vi "_PC_DataChrom_Mass2XIC.vi"(5 "ChromType":enum16{"TIC", "XIC"}(ring), 7 "Limit":T1, 8 "error in (no error)":errorcluster, 11 "File Path Array":path[](array[path])) -> (0 "error out":errorcluster, 1 "Information":string[](array[string]), 3 "DataArray":cluster{"X":dbl[], "Y":dbl[]}[](array[cluster]))   [LabVIEW 2018]
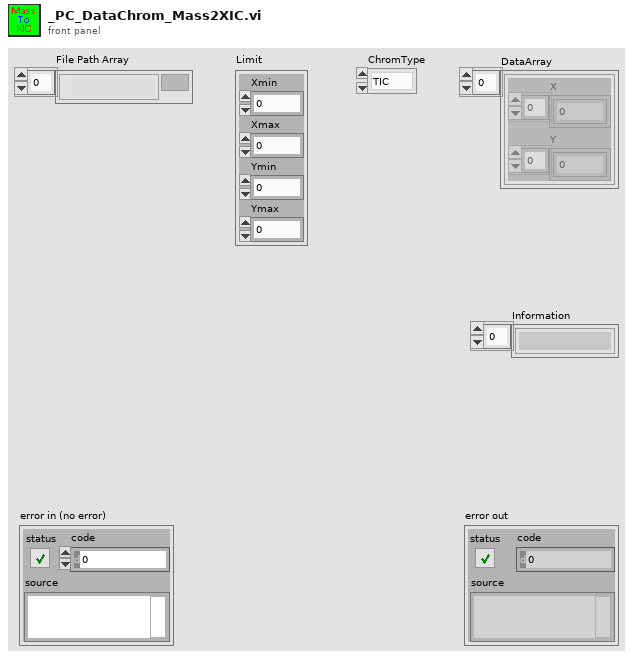
[diagram p1: front panel]
types:
  T1 = cluster{"Xmin":dbl, "Xmax":dbl, "Ymin":dbl, "Ymax":dbl}
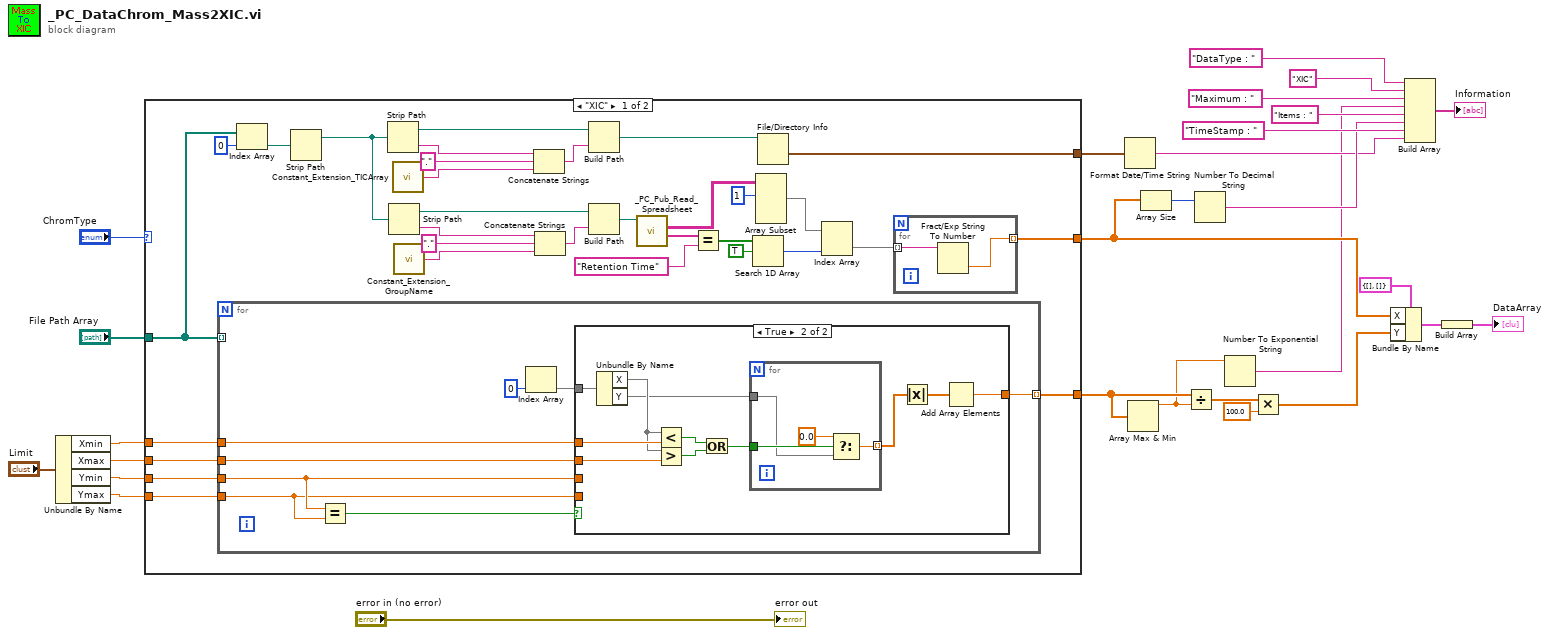
[diagram p0: block diagram]
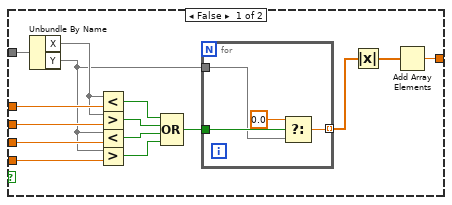
[diagram p2: hidden frame]
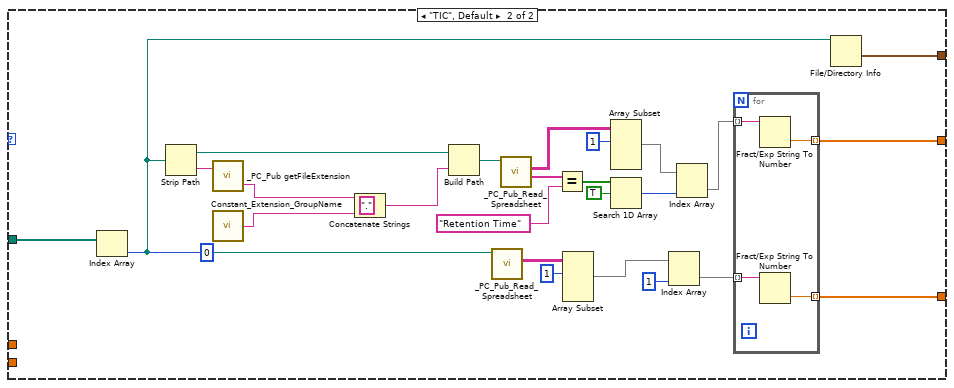
[diagram p3: hidden frame]
diagram:
  n1 = Unbundle By Name("Limit") -> ("Xmin"=w26:dbl, "Xmax"=w25:dbl, "Ymin"=w24:dbl, "Ymax"=w23:dbl)
  n2 = case shown="\"XIC\"" "ChromType" {
    tunnel: [w56 w109] -> w6
    tunnel: w26 -> [w60 _]
    tunnel: w25 -> [w59 _]
    tunnel: w24 -> [w58 _]
    tunnel: w23 -> [w57 _]
    tunnel: [w29 w110] -> w15
    tunnel: [w46 w113] -> w10
    tunnel: "File Path Array" -> [w55 w132]
    frame "XIC" {
      n3 = for {
        tunnel: [w69] -> w56 mode=indexing
        tunnel: w60 -> [w71]
        tunnel: w59 -> [w70]
        tunnel: w58 -> [w68]
        tunnel: w57 -> [w67]
        tunnel: w55 -> [_] mode=indexing
        n4 = Equal?(x=w68, y=w67) -> (x = y?=w66:bool)
        n5 = Index Array(index=0) -> (array=w65:cluster{"X":dbl[], "Y":sgl[]}[], element=w63)
        n6 = case shown="True" w66 {
          tunnel: w71 -> [w86 w101]
          tunnel: w70 -> [w85 w100]
          tunnel: w68 -> [w84 _]
          tunnel: w67 -> [w83 _]
          tunnel: [w73 w99] -> w69
          tunnel: w63 -> [w72 w91]
          frame False {
            n7 = Unbundle By Name(w72) -> ("X"=w82, "Y"=w76)
            n8 = Less?(x=w82, y=w86) -> (x < y?=w81:bool)
            n9 = Greater?(x=w82, y=w85) -> (0:w80:bool)
            n10 = Less?(x=w76, y=w84) -> (x < y?=w79:bool)
            n11 = Greater?(x=w76, y=w83) -> (0:w78:bool)
            n12 = Compound Arithmetic op=OR(w81, w80, w79, w78) -> (w77:bool)
            n13 = for {
              tunnel: w77 -> [w90]
              tunnel: w76 -> [w88]
              tunnel: [w87] -> w74 mode=indexing
              n14 = Select(t=0.0, s=w90, f=w88) -> (s? t:f=w87:dbl)
            }
            n15 = Absolute Value(x=w74) -> (abs(x)=w75:dbl[])
            n16 = Add Array Elements(numeric array=w75) -> (sum=w73:dbl)
          }
          frame True {
            n17 = Unbundle By Name(w91) -> ("X"=w98, "Y"=w94)
            n18 = Less?(x=w98, y=w101) -> (x < y?=w97:bool)
            n19 = Greater?(x=w98, y=w100) -> (0:w96:bool)
            n20 = Or(x=w97, y=w96) -> (x .or. y?=w95:bool)
            n21 = for {
              tunnel: w95 -> [w105]
              tunnel: w94 -> [w103]
              tunnel: [w102] -> w92 mode=indexing
              n22 = Select(t=0.0, s=w105, f=w103) -> (s? t:f=w102:dbl)
            }
            n23 = Absolute Value(x=w92) -> (abs(x)=w93:dbl[])
            n24 = Add Array Elements(numeric array=w93) -> (sum=w99:dbl)
          }
        }
      }
      n25 = Index Array(array=w55, index=0) -> (element=w53:path)
      n26 = Strip Path(path=w53) -> (stripped path=w33:path)  [unwired: 1 out]
      n27 = Strip Path(path=w33) -> (stripped path=w49:path, name=w50:string)
      n28 = Strip Path(path=w33) -> (stripped path=w32:path, name=w34:string)
      n29 = call "Constant_Extension_TICArray.vi"() -> ("Information Array Name String"=w51:string)
      n30 = call "Constant_Extension_GroupName.vi"() -> ("Group Name String"=w35:string)
      n31 = Concatenate Strings(w50, "." ("string"), w51) -> (w48:string)
      n32 = Concatenate Strings(w34, "." ("string"), w35) -> (w31:string)
      n33 = Build Path(base path=w49, name or relative path=w48) -> (appended path=w47:path)
      n34 = Build Path(base path=w32, name or relative path=w31) -> (appended path=w45:path)
      n35 = call "_PC_Pub_Read_Spreadsheet.vi"("file path (dialog if empty)"=w45) -> ("first row"=w39:string[], "all rows"=w38:string[][])  [unwired: 7 in, 2 out]
      n36 = Equal?(x=w39, y="Retention Time" ("String")) -> (x = y?=w43:bool[])
      n37 = Search 1D Array(1D array=w43, element=TRUE) -> (index of element=w37:i32)  [unwired: 1 in]
      n38 = Array Subset(array=w38, index (row)=1 ("index")) -> (w40:string[][])  [unwired: 3 in]
      n39 = File/Directory Info(path=w47) -> (last mod=w46:timestamp)  [unwired: 1 in, 6 out]
      n40 = Index Array(array=w40, index (col)=w37) -> (element=w30:string[])  [unwired: 1 in]
      n41 = for {
        tunnel: w30 -> [w62] mode=indexing
        tunnel: [w61] -> w29 mode=indexing
        n42 = Fract/Exp String To Number(string=w62) -> (number=w61:dbl)  [unwired: 3 in, 1 out]
      }
    }
    frame "TIC", Default {
      n43 = Index Array(array=w132, index=0) -> (element=w114:path)
      n44 = Strip Path(path=w114) -> (stripped path=w124:path, name=w126:string)
      n45 = call "_PC_Pub getFileExtension.vi"("Input"=w126) -> ("FileName"=w129:string)  [unwired: 1 in, 1 out]
      n46 = call "Constant_Extension_GroupName.vi"() -> ("Group Name String"=w127:string)
      n47 = Concatenate Strings(w129, "." ("string"), w127) -> (w125:string)
      n48 = Build Path(base path=w124, name or relative path=w125) -> (appended path=w123:path)
      n49 = call "_PC_Pub_Read_Spreadsheet.vi"("file path (dialog if empty)"=w114) -> ("all rows"=w108:string[][])  [unwired: 7 in, 3 out]
      n50 = call "_PC_Pub_Read_Spreadsheet.vi"("file path (dialog if empty)"=w123) -> ("first row"=w117:string[], "all rows"=w116:string[][])  [unwired: 7 in, 2 out]
      n51 = Equal?(x=w117, y="Retention Time" ("String")) -> (x = y?=w121:bool[])
      n52 = Array Subset(array=w108, index (row)=1 ("index")) -> (w107:string[][])  [unwired: 3 in]
      n53 = Array Subset(array=w116, index (row)=1 ("index")) -> (w118:string[][])  [unwired: 3 in]
      n54 = Search 1D Array(1D array=w121, element=TRUE) -> (index of element=w115:i32)  [unwired: 1 in]
      n55 = Index Array(array=w107, index (col)=1 ("disabled index (col)")) -> (element=w112:string[])  [unwired: 1 in]
      n56 = Index Array(array=w118, index (col)=w115) -> (element=w111:string[])  [unwired: 1 in]
      n57 = for {
        tunnel: w112 -> [w135] mode=indexing
        tunnel: w111 -> [w136] mode=indexing
        tunnel: [w134] -> w109 mode=indexing
        tunnel: [w133] -> w110 mode=indexing
        n58 = Fract/Exp String To Number(string=w136) -> (number=w133:dbl)  [unwired: 3 in, 1 out]
        n59 = Fract/Exp String To Number(string=w135) -> (number=w134:dbl)  [unwired: 3 in, 1 out]
      }
      n60 = File/Directory Info(path=w114) -> (last mod=w113:timestamp)  [unwired: 1 in, 6 out]
    }
  }
  n61 = Format Date/Time String(seconds (now)=w10) -> (date/time string=w9:string)  [unwired: 2 in]
  n62 = Array Max & Min(array=w6) -> (max value=w5:dbl)  [unwired: 3 out]
  n63 = Array Size(array=w15) -> (size(s)=w13:i32)
  n64 = Divide(x=w6, y=w5) -> (x/y=w8:dbl[])
  n65 = Number To Decimal String(number=w13) -> (decimal integer string=w12:string)  [unwired: 1 in]
  n66 = Number To Exponential String(number=w5) -> (E-format string=w4:string)  [unwired: 3 in]
  n67 = Multiply(x=w8, y=100.0) -> (x*y=w3:dbl[])
  n68 = Bundle By Name(cluster=cluster{"X":dbl[], "Y":dbl[]} {"X"=[], "Y"=[]} ("Data"), "X"=w15, "Y"=w3) -> (w2:cluster{"X":dbl[], "Y":dbl[]})
  n69 = Build Array("DataType : ", "XIC", "Maximum : ", w4, "Items : ", w12, "TimeStamp : ", w9) -> (→"Information":string[])
  n70 = Build Array(w2) -> (→"DataArray":cluster{"X":dbl[], "Y":dbl[]}[])
  "error out" <- "error in (no error)"
